vi "Unit Test.vi"() -> ()   [LabVIEW 2018]
uses:
  PPLs/Laser/Parent/Laser.lvlibp/Custom Controls/Laser Type.ctl
  Gen 2.lvclass
  PPLs/Laser/Parent/Laser.lvlibp/Laser.lvclass
  C:/Projects/LabVIEW/PPLs/Laser/Parent/Laser.lvlibp/Laser.lvclass
panel:
  in  "AutoScroll?":bool
  out "Buffer":string
  in  "Read Buffer":bool
  in  "Send Commands":bool
  in  "Commands":string[](array[string])
  out "error out":errorcluster
  in  "stop":bool
  in  "Resource":refnum<visa-resource-name>
  in  "error in (no error)":errorcluster
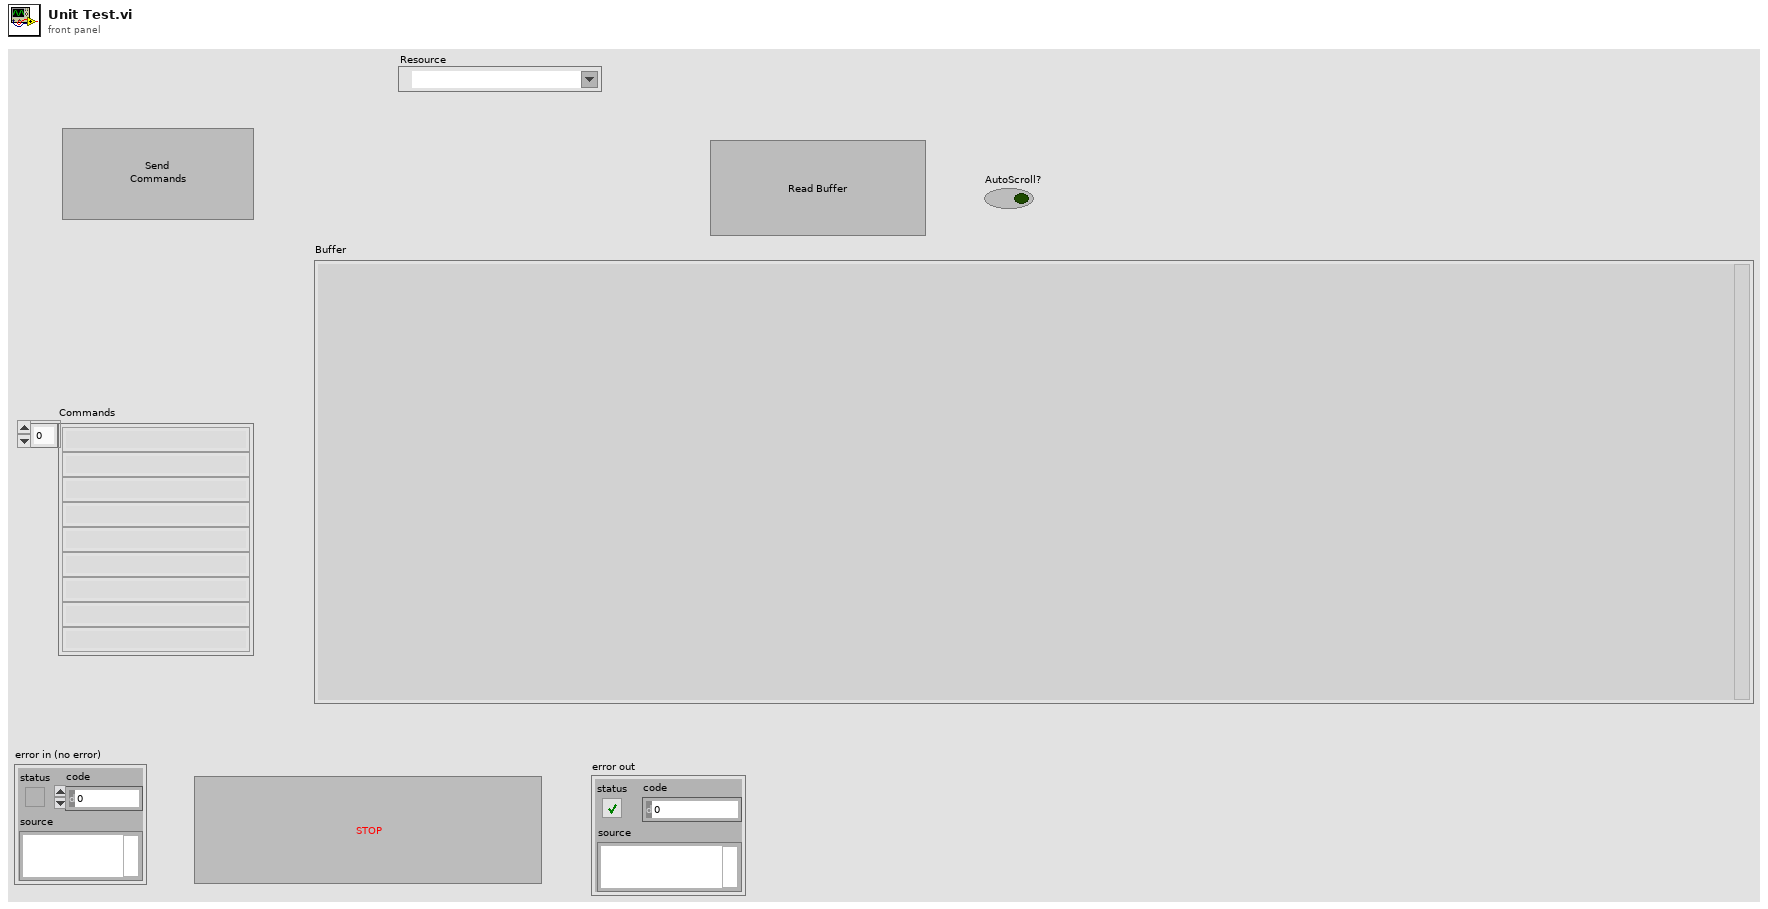
[diagram p1: front panel]
types:
  T1 = typedef "Laser.lvlibp/Laser.lvclass/Laser Type.ctl" = enum16{"Model H", "Model I"}
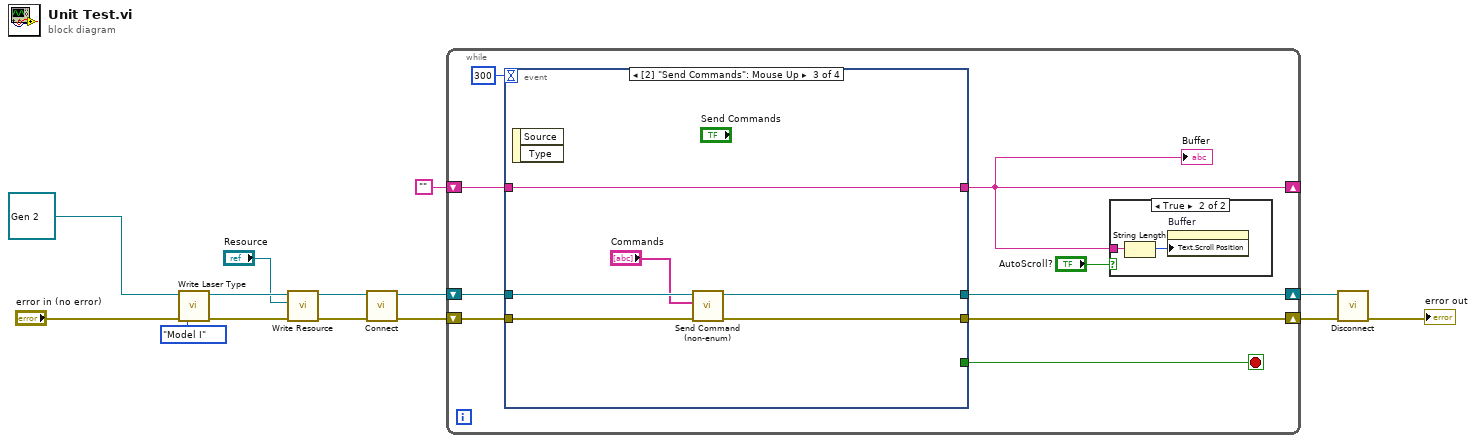
[diagram p0: block diagram]
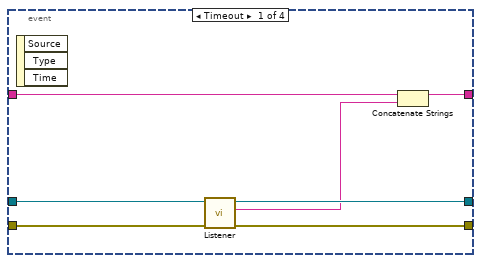
[diagram p3: hidden frame]
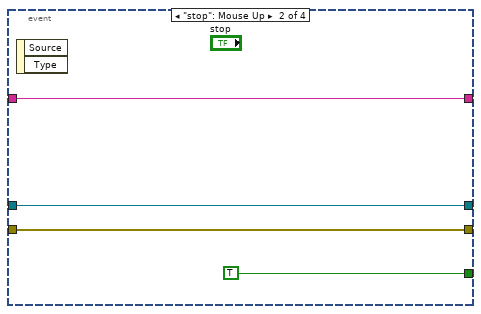
[diagram p4: hidden frame]
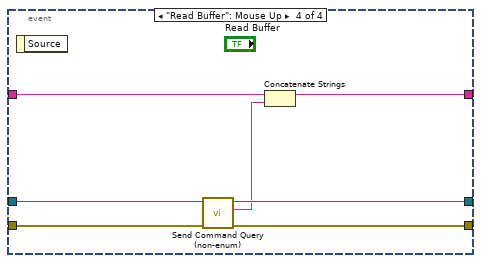
[diagram p5: hidden frame]
diagram:
  n1 = call "Write Laser Type .vi"("error in (no error)"="error in (no error)", "Laser Type"=Laser_Type."Model I", "Laser in"=refnum<class "Gen 2.lvclass"> refnum ("Gen 2.lvlib:Gen 2.lvclass")) -> ("error out"=w10:errorcluster, "Laser out"=w11:refnum<class "Gen 2.lvclass">)  [unwired: 7 in]
  n2 = call "Write Resource.vi"("error in (no error)"=w10, "Resource"="Resource", "Laser in"=w11) -> ("error out"=w7:errorcluster, "Laser out"=w8:refnum<class "Gen 2.lvclass">)  [unwired: 7 in]
  n3 = call-dynamic "Connect.vi"("error in (no error)"=w7, "Gen 2 in"=w8) -> ("error out"=w5:errorcluster, "Gen 2 out"=w6:refnum<class "Gen 2.lvclass">)  [unwired: 8 in]
  n4 = while {
    shift-right: [w22] -> w4
    shift-left: w6 -> [w21]
    shift-right: [w20] -> w3
    shift-left: w5 -> [w19]
    shift-right: [w16] -> _
    shift-left: "" -> [w17]
    stop <- w23 stop-if-true
    n5 = event shown="[2] \"Send Commands\": Mouse Up" {
      selector: _ -> [_ _ _ _]
      dyn-events: _ -> [_ _ _ _]
      timeout: 300 -> [_ _ _ _]
      tunnel: [_ TRUE _ _] -> w23
      tunnel: [w28 w35 w39 w47] -> w22
      tunnel: w21 -> [w30 w35 w42 w49]
      tunnel: [w26 w34 w38 w46] -> w20
      tunnel: w19 -> [w29 w34 w41 w48]
      tunnel: [w31 w33 w37 w43] -> w16
      tunnel: w17 -> [w32 w33 w37 w45]
      event Timeout {
        n6 = event-data() -> ()  [unwired: 1 in, 3 out]
        n7 = call-dynamic "Listener.vi"("error in (no error)"=w29, "Gen 2 in"=w30) -> ("error out"=w26:errorcluster, "Buffer Dump"=w27:string, "Gen 2 out"=w28:refnum<class "Gen 2.lvclass">)  [unwired: 7 in]
        n8 = Concatenate Strings(w32, w27) -> (w31:string)
      }
      event "stop": Mouse Up {
        n9 = event-data() -> ()  [unwired: 1 in, 2 out]
      }
      event "Send Commands": Mouse Up {
        n10 = event-data() -> ()  [unwired: 1 in, 2 out]
        n11 = call-dynamic "Send Command (non-enum).vi"("error in (no error)"=w41, "Commands"="Commands", "Gen 2 in"=w42) -> ("error out"=w38:errorcluster, "Gen 2 out"=w39:refnum<class "Gen 2.lvclass">)  [unwired: 7 in]
      }
      event "Read Buffer": Mouse Up {
        n12 = event-data() -> ()  [unwired: 1 in, 1 out]
        n13 = call-dynamic "Send Command Query (non-enum).vi"("error in (no error)"=w48, "Gen 2 in"=w49) -> ("error out"=w46:errorcluster, "Response"=w44:string, "Gen 2 out"=w47:refnum<class "Gen 2.lvclass">)  [unwired: 7 in]
        n14 = Concatenate Strings(w45, w44) -> (w43:string)
      }
    }
    "Buffer" <- w16
    n15 = case shown="True" "AutoScroll?" {
      tunnel: w16 -> [_ w25]
      frame False {
      }
      frame True {
        n16 = String Length(string=w25) -> (length=w24:i32)
        n17 = property on="Buffer" class="Str"("Text.Scroll Position"=w24) -> ()  [unwired: 2 in, 2 out]
      }
    }
  }
  n18 = call-dynamic "Disconnect.vi"("error in"=w3, "Gen 2 in"=w4) -> ("error out"=→"error out":errorcluster)  [unwired: 8 in, 1 out]
